vi "Autonomous Independent.vi"() -> ()   [LabVIEW 2014]
doc: "This VI is called when autonomous begins, and will automatically be terminated when autonomous ends. You can carry out timed or sensor driven robot movement independently without needing to return to the caller."
uses:
  Robot Global Data.vi
  <vilib>/Rock Robotics/WPI/Solenoid/Deprecated/WPI_SolenoidSetBool.vi
  <vilib>/Rock Robotics/WPI/DriverStation/DriverStationLCD/WPI_DriverStationLCDLCDLine.ctl
  <vilib>/Rock Robotics/SystemInterfaces/Typedef/FPGA_TypedefAnalogModule.ctl
  <vilib>/Rock Robotics/SystemInterfaces/AI/FPGA_AIChannel.ctl
  <vilib>/Rock Robotics/WPI/Gyro/WPI_GyroDevRef.ctl
panel:
  out "Boolean":bool
  in  "error in (no error)":errorcluster
  in  "GyroDevRef":T1={"DevStatus"={"status"=FALSE, "code"=0, "source"=""}, "Analog Module"=enum."Controller 1", "Analog Channel"=enum."AI 1", "Offset"=0.0, "Gain (VoltsPerDegree/Second)"=0.0}
  out "Gyro":dbl=111.9833474371419
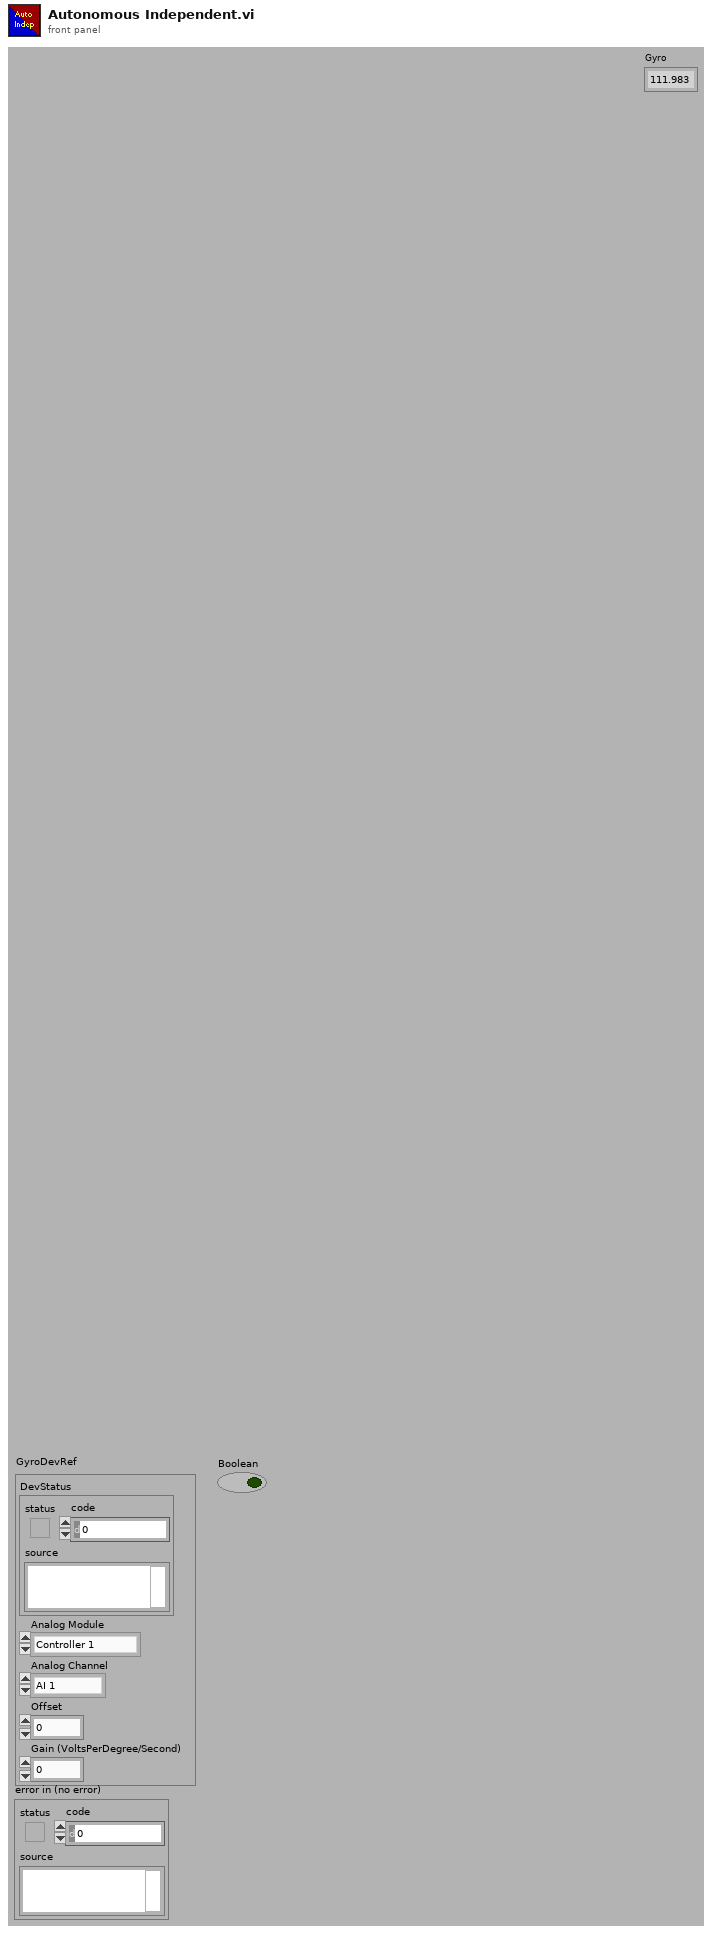
[diagram p1: front panel]
types:
  T1 = typedef "WPI_GyroDevRef.ctl" = cluster{"DevStatus":errorcluster, "Analog Module":T2, "Analog Channel":T3, "Offset":dbl, "Gain (VoltsPerDegree/Second)":dbl}
  T2 = typedef "FPGA_TypedefAnalogModule.ctl" = enum16{"Controller 1"}
  T3 = typedef "FPGA_AIChannel.ctl" = enum8{"AI 0", "AI 1", "AI 2", "AI 3", "AI MXP 0", "AI MXP 1", "AI MXP 2", "AI MXP 3", "Invalid"}
  T4 = typedef "WPI_DriverStationLCDLCDLine.ctl" = enum16{"Main - Line 1", "User - Line 2", "User - Line 3", "User - Line 4", "User - Line 5", "User - Line 6"}
  T5 = cluster{"Digital Input [1-16][0]":bool, "Digital Input [1-16][1]":bool, "Digital Input [1-16][2]":bool, "Digital Input [1-16][3]":bool, "Digital Input [1-16][4]":bool, "Digital Input [1-16][5]":bool, "Digital Input [1-16][6]":bool, "Digital Input [1-16][7]":bool, "Digital Input [1-16][8]":bool, "Digital Input [1-16][9]":bool, "Digital Input [1-16][10]":bool, "Digital Input [1-16][11]":bool, "Digital Input [1-16][12]":bool, "Digital Input [1-16][13]":bool, "Digital Input [1-16][14]":bool, "Digital Input [1-16][15]":bool}
  T6 = typedef "WPI_GyroDevRef.ctl" = cluster{"DevStatus":errorcluster, "Analog Module":T7, "Analog Channel":T8, "Offset":dbl, "Gain (VoltsPerDegree/Second)":dbl}
  T7 = typedef "FPGA_TypedefAnalogModule.ctl" = enum16{"Analog Module 1", "Analog Module 2"}
  T8 = typedef "FPGA_AIChannel.ctl" = enum8{"AI 1", "AI 2", "AI 3", "AI 4", "AI 5", "AI 6", "AI 7", "AI 8", "Invalid"}
  T9 = typedef "WPI_SolenoidDevRef.ctl" = cluster{"DevStatus":errorcluster, "Solenoid Module":T10, "Forward Solenoid Channel":T11, "Reverse Solenoid Channel":T11}
  T10 = typedef "FPGA_TypedefSolenoidModule.ctl" = enum16{"Solenoid Module 1", "Solenoid Module 2"}
  T11 = typedef "WPI_SolenoidChannel.ctl" = enum8{"Solenoid 1", "Solenoid 2", "Solenoid 3", "Solenoid 4", "Solenoid 5", "Solenoid 6", "Solenoid 7", "Solenoid 8", "Invalid"}
  T12 = typedef "WPI_EncoderDevRef.ctl" = cluster{"DevStatus":errorcluster, "EncoderIndex":T13, "CounterIndex":T14, "DistancePerCount":dbl, "Decoding Type":T15}
  T13 = typedef "FPGA_EncoderIdx.ctl" = enum8{"Enc 0", "Enc 1", "Enc 2", "Enc 3", "Invalid"}
  T14 = typedef "FPGA_CounterCtrSystemIndex.ctl" = enum8{"Ctr 0", "Ctr 1", "Ctr 2", "Ctr 3", "Ctr 4", "Ctr 5", "Ctr 6", "Ctr 7", "Invalid"}
  T15 = typedef "WPI_EncoderType.ctl" = enum16{"1x", "2x", "4x"}
  T16 = typedef "WPI_JoystickDevRef.ctl" = cluster{"Device":T17}
  T17 = typedef "WPI_JoystickDeviceEnum.ctl" = enum16{"USB 1", "USB 2", "USB 3", "USB 4", "Kinect 1", "Kinect 2"}
  T18 = typedef "WPI_JoystickButtonState.ctl" = cluster{"Button 1":bool, "Button 2":bool, "Button 3":bool, "Button 4":bool, "Button 5":bool, "Button 6":bool, "Button 7":bool, "Button 8":bool, "Button 9":bool, "Button 10":bool, "Button 11":bool, "Button 12":bool}
  T19 = typedef "WPI_DigitalInputDevRef.ctl" = cluster{"DevStatus":errorcluster, "DIO Channel":T20, "Digital Module":T21}
  T20 = typedef "FPGA_DIOChannel.ctl" = enum8{"DIO 1", "DIO 2", "DIO 3", "DIO 4", "DIO 5", "DIO 6", "DIO 7", "DIO 8", "DIO 9", "DIO 10", "DIO 11", "DIO 12", "DIO 13", "DIO 14", "Invalid"}
  T21 = typedef "FPGA_TypedefDigitalModule.ctl" = enum16{"Digital Module 1", "Digital Module 2"}
  T22 = typedef "WPI_RobotDriveDevRef.ctl" = cluster{"DevStatus":errorcluster, "Motors[]":T23[], "Square Inputs":bool, "Max Output":dbl, "Isochronous":bool}
  T23 = typedef "WPI_MotorControlDeviceRef.ctl" = cluster{"DeviceStatus":errorcluster, "Type":enum16{"PWM", "CAN"}, "PWM":cluster{"Digital Module":T21, "PWM Channel":T24, "DeadBand":T25}, "CAN":cluster{"Device Number":u8, "Control Mode":T26, "Semaphore":T27, "Max Vout":dbl}, "Invert":bool, "TransformRef":T28, "InvTransformRef":T28}
  T24 = typedef "FPGA_DIOPWMChannel.ctl" = enum8{"PWM 1", "PWM 2", "PWM 3", "PWM 4", "PWM 5", "PWM 6", "PWM 7", "PWM 8", "PWM 9", "PWM 10", "Invalid"}
  T25 = typedef "WPI_PWMDeadband.ctl" = cluster{"Name":string, "maxPositivePwm":i32, "minPositivePwm":i32, "centerPwm":i32, "maxNegativePwm":i32, "minNegativePwm":i32, "angularRange":u16}
  T26 = typedef "WPI_CANJaguar_ControlMode.ctl" = enum8{"Percent VBus", "Current", "Speed", "Position", "Voltage"}
  T27 = typedef "Semaphore RefNum" = refnum<k1>
  T28 = typedef "WPI_PWMTransform_ConPane.ctl" = refnum<vi>
  T29 = cluster{"axis 1 (x)":dbl, "axis 2 (y)":dbl, "axis 3 (throttle)":dbl, "axis 4":dbl, "axis 5":dbl, "axis 6":dbl}
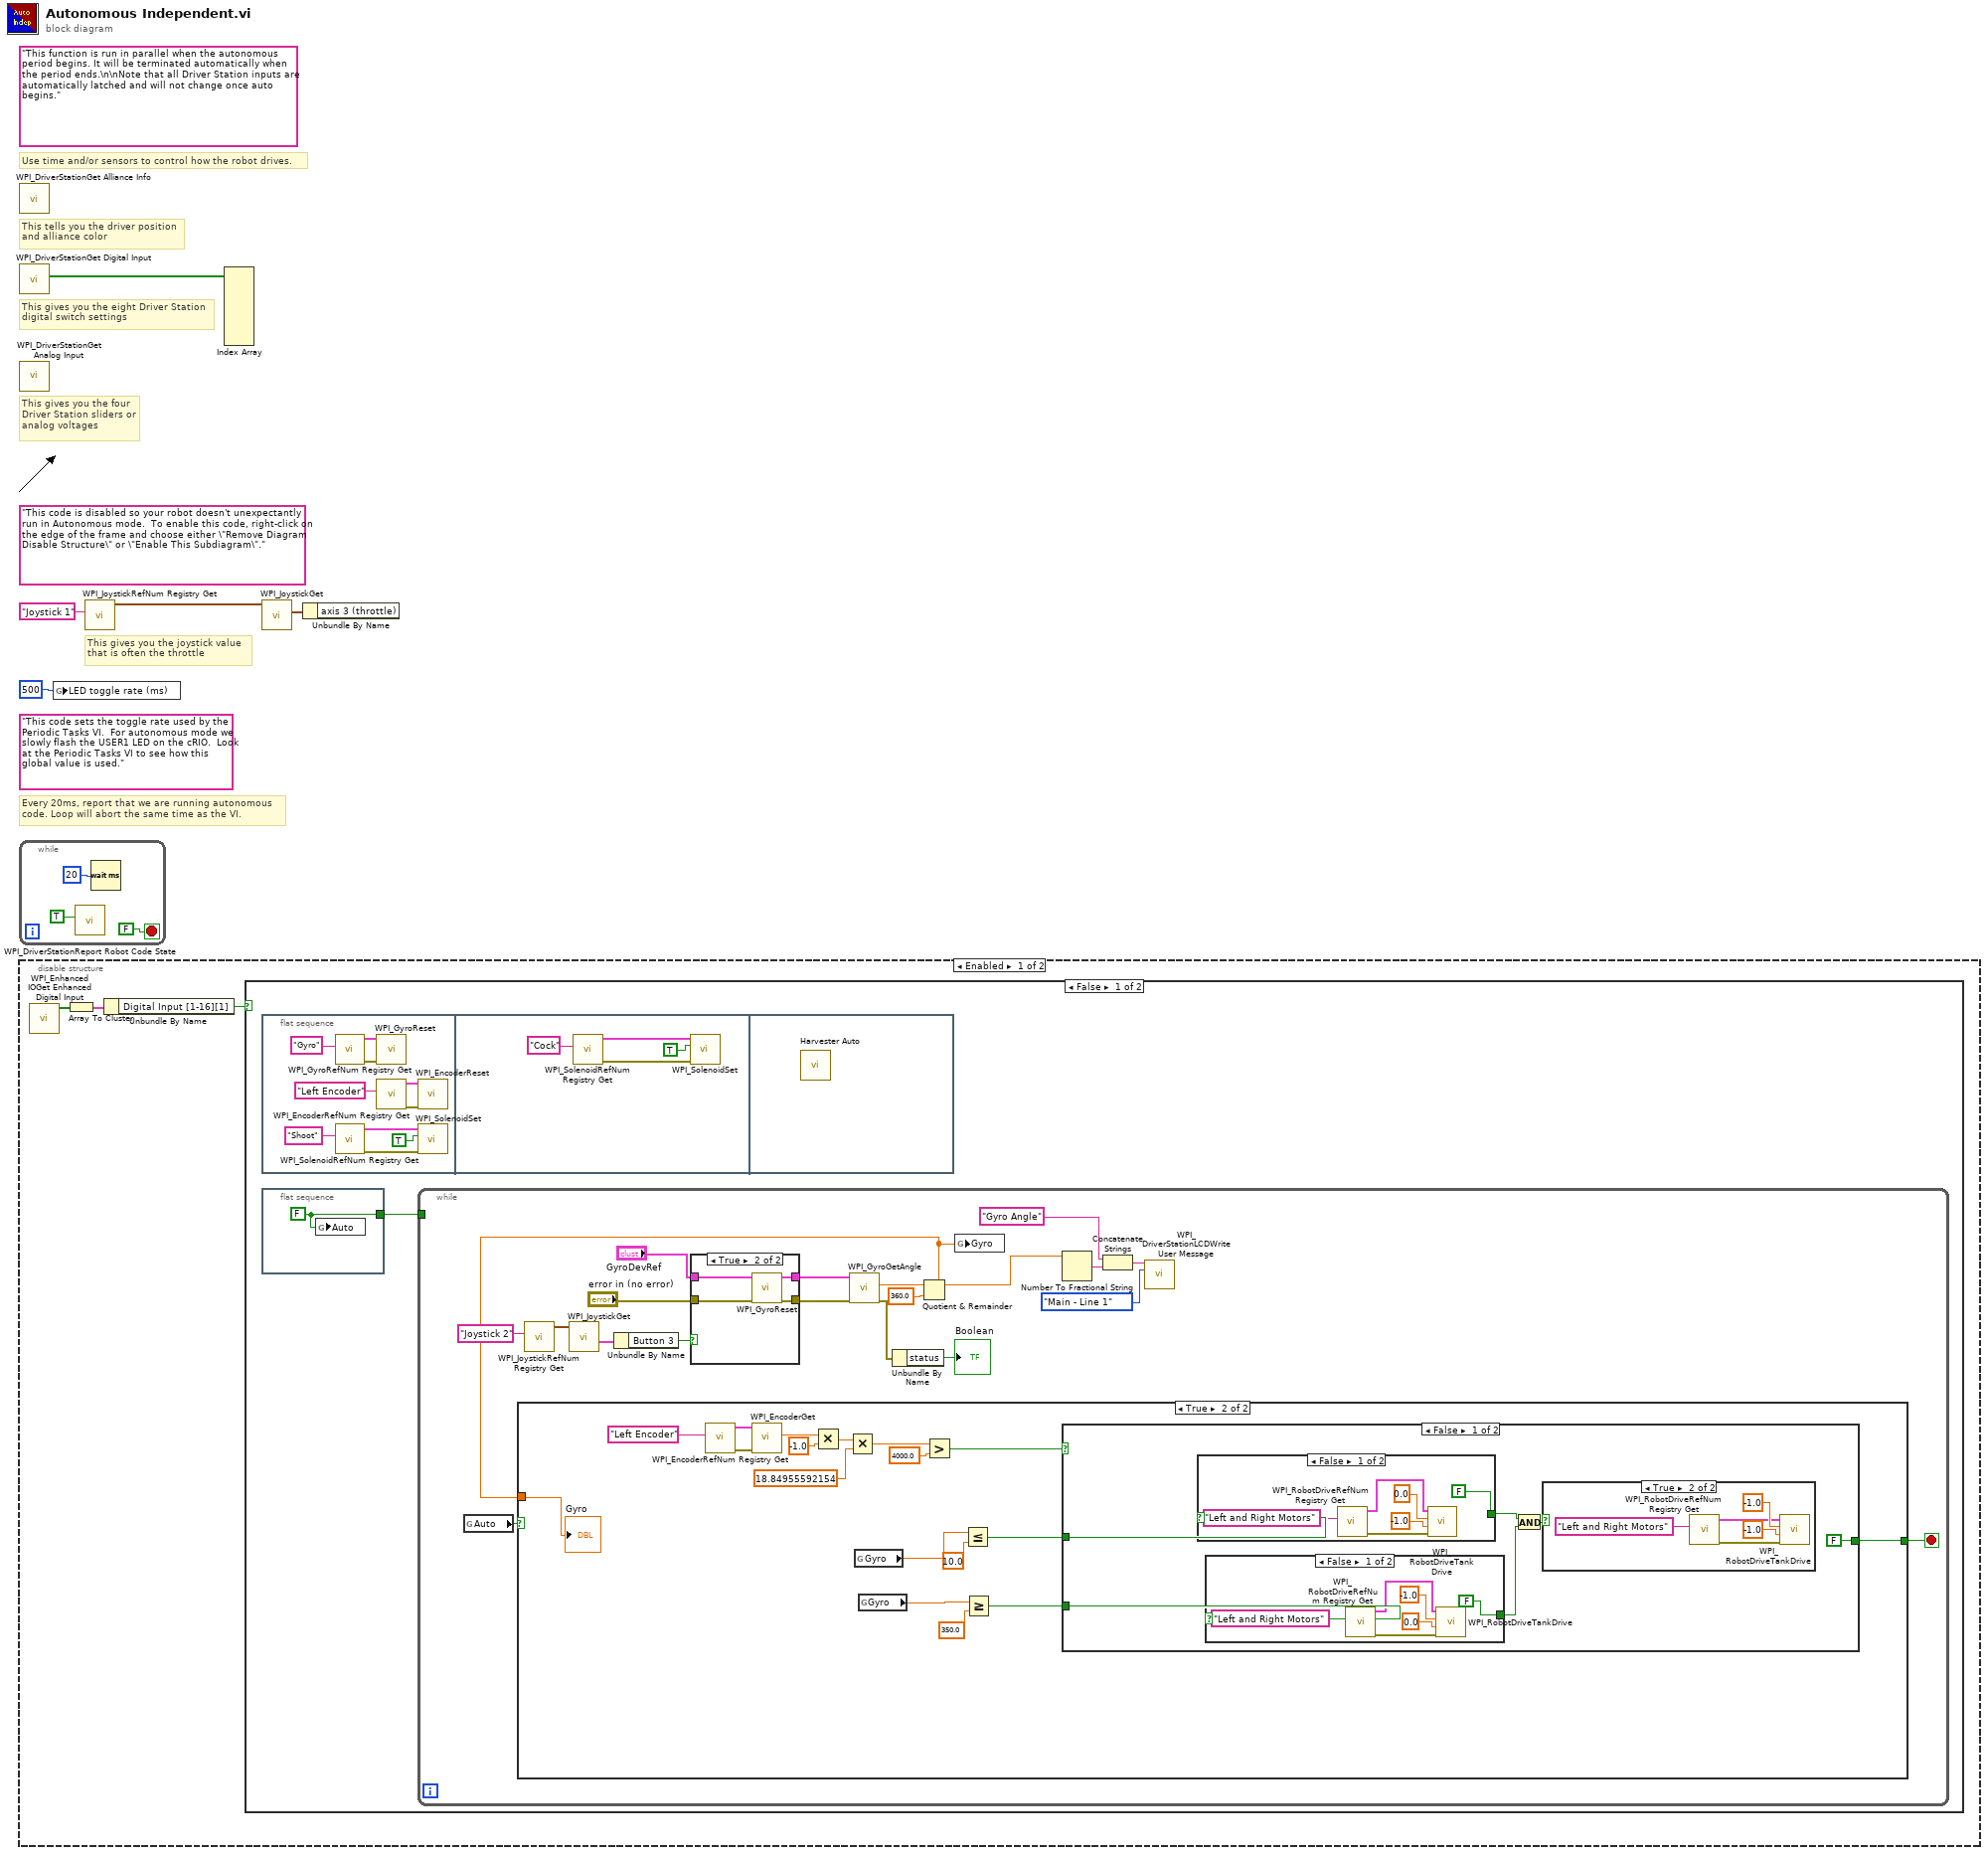
[diagram p0: block diagram]
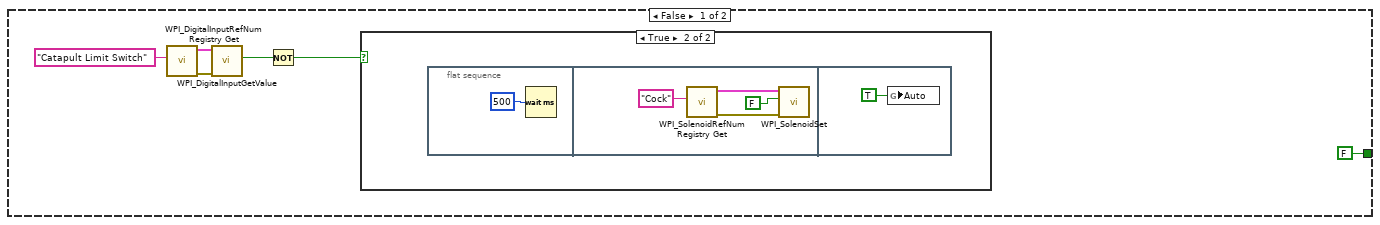
[diagram p3: hidden frame]
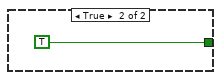
[diagram p6: hidden frame]
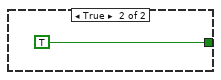
[diagram p7: hidden frame]
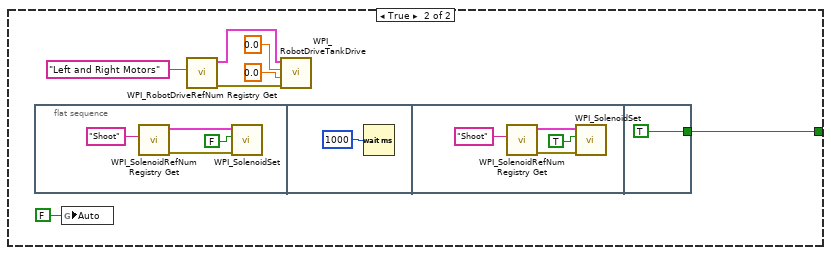
[diagram p8: hidden frame]
diagram:
  (unwired) "This code sets the toggle rate used by the Periodic Tasks VI.  For autonomous mode we slowly flash the USER1 LED on the cRIO.  Look at the Periodic Tasks VI to see how this global value is used."
  (unwired) "This code is disabled so your robot doesn't unexpectantly run in Autonomous mode.  To enable this code, right-click on the edge of the frame and choose either \"Remove Diagram Disable Structure\" or \"Enable This Subdiagram\"."
  (unwired) "This function is run in parallel when the autonomous period begins. It will be terminated automatically when the period ends.\n\nNote that all Driver Station inputs are automatically latched and will not change once auto begins."
  # "Every 20ms, report that we are running autonomous\ncode. Loop will abort the same time as the VI."
  # "This gives you the joystick value\nthat is often the throttle"
  # "Use time and/or sensors to control how the robot drives."
  # "This tells you the driver position\nand alliance color"
  # "This gives you the eight Driver Station\ndigital switch settings"
  # "This gives you the four\nDriver Station sliders or\nanalog voltages"
  n1 = call <vilib>:"WPI_DriverStationGet Alliance Info.vi"() -> ()  [unwired: 12 out]
  n2 = call <vilib>:"WPI_DriverStationGet Digital Input.vi"() -> ("Driver Station Digital Input (1-8)"=w5:bool[])  [unwired: 11 out]
  n3 = call <vilib>:"WPI_DriverStationGet Analog Input.vi"() -> ()  [unwired: 12 out]
  n4 = while {
    stop <- FALSE stop-if-true
    n5 = call <vilib>:"WPI_DriverStationReport Robot Code State.vi"("Autonomous"=TRUE) -> ()  [unwired: 10 in, 1 out]
    n6 = Wait (ms)(milliseconds to wait=u32 20) -> ()  [unwired: 1 out]
  }
  n7 = disable-structure shown="Enabled" {
    frame Enabled {
      n8 = call <vilib>:"WPI_Enhanced IOGet Enhanced Digital Input.vi"() -> ("Digital Input [1-16]"=w11:bool[])  [unwired: 10 in, 1 out]
      n9 = Array To Cluster(array=w11) -> (cluster=w10:T5)
      n10 = Unbundle By Name(w10) -> ("Digital Input [1-16][1]"=w9:bool)
      n11 = case shown="False" w9 {
        frame False {
          n12 = flat-sequence {
            frame #0 {
              n13 = call <vilib>:"WPI_GyroRefNum Registry Get.vi"("refnum name"="Gyro") -> ("error out"=w112:errorcluster, "GyroDevRef"=w113:T6)  [unwired: 9 in]
              n14 = call <vilib>:"WPI_SolenoidRefNum Registry Get.vi"("refnum name"="Shoot") -> ("error out"=w114:errorcluster, "SolenoidDevRef"=w115:T9)  [unwired: 9 in]
              n15 = call <vilib>:"WPI_GyroReset.vi"("error in (no error)"=w112, "GyroDevRef"=w113) -> ()  [unwired: 10 out]
              n16 = call <vilib>:"WPI_EncoderRefNum Registry Get.vi"("refnum name"="Left Encoder") -> ("error out"=w120:errorcluster, "EncoderDevRef"=w119:T12)  [unwired: 9 in]
              n17 = call <vilib>:"WPI_EncoderReset.vi"("error in (no error)"=w120, "EncoderDevRef"=w119) -> ()  [unwired: 8 in, 2 out]
              n18 = call-poly <vilib>:"WPI_SolenoidSet.vi"("error in (no error)"=w114, "Value"=TRUE, "SolenoidDevRef"=w115) -> ()  [unwired: 7 in, 2 out]
            }
            frame #1 {
              n19 = call <vilib>:"WPI_SolenoidRefNum Registry Get.vi"("refnum name"="Cock") -> ("error out"=w124:errorcluster, "SolenoidDevRef"=w122:T9)  [unwired: 9 in]
              n20 = call-poly <vilib>:"WPI_SolenoidSet.vi"("error in (no error)"=w124, "Value"=TRUE, "SolenoidDevRef"=w122) -> ()  [unwired: 7 in, 2 out]
            }
            frame #2 {
              n21 = call "Harvester Auto.vi"() -> ()  [unwired: 12 in]
            }
          }
          n22 = flat-sequence {
            tunnel: [w13] -> w12
            frame #0 {
              w13 = FALSE
              n23 = global write "Robot Global Data.vi" "Auto"(w13) -> ()
            }
          }
          n24 = while {
            tunnel: w12 -> [_]
            stop <- w31 stop-if-true
            n25 = global read "Robot Global Data.vi" "Auto"() -> (w32:bool)
            n26 = call <vilib>:"WPI_JoystickRefNum Registry Get.vi"("refnum name"="Joystick 2") -> ("JoystickDevRef"=w28:T16)  [unwired: 1 in, 9 out]
            n27 = call <vilib>:"WPI_JoystickGet.vi"("JoystickDevRef"=w28) -> ("Buttons"=w29:T18)  [unwired: 1 in, 5 out]
            n28 = Unbundle By Name(w29) -> ("Button 3"=w30:bool)
            n29 = case shown="True" w30 {
              tunnel: [w34 w38] -> w20
              tunnel: [w33 w37] -> w23
              tunnel: "GyroDevRef" -> [w34 w36]
              tunnel: "error in (no error)" -> [w33 w35]
              frame False {
              }
              frame True {
                n30 = call <vilib>:"WPI_GyroReset.vi"("error in (no error)"=w35, "GyroDevRef"=w36) -> ("error out"=w37:errorcluster, "GyroDevRef"=w38:T6)  [unwired: 8 out]
              }
            }
            n31 = call <vilib>:"WPI_GyroGetAngle.vi"("error in (no error)"=w23, "GyroDevRef"=w20) -> ("error out"=w21:errorcluster, "Angle"=w16:dbl)  [unwired: 8 out]
            n32 = Unbundle By Name(w21) -> ("status"=→"Boolean":bool)
            n33 = Quotient & Remainder(x=w16, y=360.0) -> (x-y*floor(x/y)=w14:dbl)  [unwired: 1 out]
            n34 = case shown="True" w32 {
              tunnel: [FALSE w59] -> w31
              tunnel: w14 -> [_ w57]
              frame False {
                n35 = call <vilib>:"WPI_DigitalInputRefNum Registry Get.vi"("refnum name"="Catapult Limit Switch") -> ("error out"=w40:errorcluster, "DigitalInputDevRef"=w41:T19)  [unwired: 9 in]
                n36 = call <vilib>:"WPI_DigitalInputGetValue.vi"("error in (no error)"=w40, "DigitalInputDevRef"=w41) -> ("Value"=w43:bool)  [unwired: 7 in, 2 out]
                n37 = Not(x=w43) -> (.not. x?=w42:bool)
                n38 = case shown="True" w42 {
                  frame False {
                  }
                  frame True {
                    n39 = flat-sequence {
                      frame #0 {
                        n40 = Wait (ms)(milliseconds to wait=u32 500) -> ()  [unwired: 1 out]
                      }
                      frame #1 {
                        n41 = call <vilib>:"WPI_SolenoidRefNum Registry Get.vi"("refnum name"="Cock") -> ("error out"=w46:errorcluster, "SolenoidDevRef"=w47:T9)  [unwired: 9 in]
                        n42 = call-poly <vilib>:"WPI_SolenoidSet.vi"("error in (no error)"=w46, "Value"=FALSE, "SolenoidDevRef"=w47) -> ()  [unwired: 7 in, 2 out]
                      }
                      frame #2 {
                        n43 = global write "Robot Global Data.vi" "Auto"(TRUE) -> ()
                      }
                    }
                  }
                }
              }
              frame True {
                n44 = call <vilib>:"WPI_EncoderRefNum Registry Get.vi"("refnum name"="Left Encoder") -> ("error out"=w62:errorcluster, "EncoderDevRef"=w61:T12)  [unwired: 9 in]
                n45 = call <vilib>:"WPI_EncoderGet.vi"("error in (no error)"=w62, "EncoderDevRef"=w61) -> ("Distance"=w64:dbl)  [unwired: 4 in, 5 out]
                n46 = Multiply(x=w64, y=-1.0) -> (x*y=w63:dbl)
                n47 = Multiply(x=w63, y=18.84955592154) -> (x*y=w60:dbl)
                n48 = global read "Robot Global Data.vi" "Gyro"() -> (w55:dbl)
                n49 = global read "Robot Global Data.vi" "Gyro"() -> (w53:dbl)
                n50 = Greater?(x=w60, y=4000.0) -> (0:w58:bool)
                n51 = Less Or Equal?(x=w55, y=10.0) -> (x <= y?=w52:bool)
                n52 = Greater Or Equal?(x=w53, y=350.0) -> (x >= y?=w51:bool)
                n53 = case shown="False" w58 {
                  tunnel: [FALSE w94] -> w59
                  tunnel: w52 -> [w73 _]
                  tunnel: w51 -> [w72 _]
                  frame False {
                    n54 = case shown="False" w73 {
                      tunnel: [FALSE TRUE] -> w70
                      frame False {
                        n55 = call <vilib>:"WPI_RobotDriveRefNum Registry Get.vi"("refnum name"="Left and Right Motors") -> ("error out"=w88:errorcluster, "RobotDriveDevRef"=w89:T22)  [unwired: 9 in]
                        n56 = call <vilib>:"WPI_RobotDriveTankDrive.vi"("error in (no error)"=w88, "Right axis value"=-1.0 ("RightSpeed"), "Left axis value"=0.0 ("LeftSpeed"), "RobotDriveDevRef"=w89) -> ()  [unwired: 5 in, 3 out]
                      }
                      frame True {
                      }
                    }
                    n57 = case shown="False" w72 {
                      tunnel: [FALSE TRUE] -> w69
                      frame False {
                        n58 = call <vilib>:"WPI_RobotDriveRefNum Registry Get.vi"("refnum name"="Left and Right Motors") -> ("error out"=w81:errorcluster, "RobotDriveDevRef"=w82:T22)  [unwired: 9 in]
                        n59 = call <vilib>:"WPI_RobotDriveTankDrive.vi"("error in (no error)"=w81, "Right axis value"=0.0 ("RightSpeed"), "Left axis value"=-1.0 ("LeftSpeed"), "RobotDriveDevRef"=w82) -> ()  [unwired: 5 in, 3 out]
                      }
                      frame True {
                      }
                    }
                    n60 = And(x=w70, y=w69) -> (x .and. y?=w71:bool)
                    n61 = case shown="True" w71 {
                      frame False {
                      }
                      frame True {
                        n62 = call <vilib>:"WPI_RobotDriveRefNum Registry Get.vi"("refnum name"="Left and Right Motors") -> ("error out"=w75:errorcluster, "RobotDriveDevRef"=w76:T22)  [unwired: 9 in]
                        n63 = call <vilib>:"WPI_RobotDriveTankDrive.vi"("error in (no error)"=w75, "Right axis value"=-1.0 ("RightSpeed"), "Left axis value"=-1.0 ("LeftSpeed"), "RobotDriveDevRef"=w76) -> ()  [unwired: 5 in, 3 out]
                      }
                    }
                  }
                  frame True {
                    n64 = flat-sequence {
                      tunnel: [TRUE] -> w94
                      frame #0 {
                        n65 = call <vilib>:"WPI_SolenoidRefNum Registry Get.vi"("refnum name"="Shoot") -> ("error out"=w104:errorcluster, "SolenoidDevRef"=w101:T9)  [unwired: 9 in]
                        n66 = call-poly <vilib>:"WPI_SolenoidSet.vi"("error in (no error)"=w104, "Value"=FALSE, "SolenoidDevRef"=w101) -> ()  [unwired: 7 in, 2 out]
                      }
                      frame #1 {
                        n67 = Wait (ms)(milliseconds to wait=u32 1000) -> ()  [unwired: 1 out]
                      }
                      frame #2 {
                        n68 = call <vilib>:"WPI_SolenoidRefNum Registry Get.vi"("refnum name"="Shoot") -> ("error out"=w109:errorcluster, "SolenoidDevRef"=w108:T9)  [unwired: 9 in]
                        n69 = call-poly <vilib>:"WPI_SolenoidSet.vi"("error in (no error)"=w109, "Value"=TRUE, "SolenoidDevRef"=w108) -> ()  [unwired: 7 in, 2 out]
                      }
                      frame #3 {
                      }
                    }
                    n70 = global write "Robot Global Data.vi" "Auto"(FALSE) -> ()
                    n71 = call <vilib>:"WPI_RobotDriveRefNum Registry Get.vi"("refnum name"="Left and Right Motors") -> ("error out"=w96:errorcluster, "RobotDriveDevRef"=w97:T22)  [unwired: 9 in]
                    n72 = call <vilib>:"WPI_RobotDriveTankDrive.vi"("error in (no error)"=w96, "Right axis value"=0.0 ("RightSpeed"), "Left axis value"=0.0 ("LeftSpeed"), "RobotDriveDevRef"=w97) -> ()  [unwired: 5 in, 3 out]
                  }
                }
                "Gyro" <- w57
              }
            }
            n73 = global write "Robot Global Data.vi" "Gyro"(w14) -> ()
            n74 = Number To Fractional String(number=w14) -> (F-format string=w18:string)  [unwired: 3 out]
            n75 = Concatenate Strings("Gyro Angle" ("string"), w18) -> (w22:string)
            n76 = call <vilib>:"WPI_DriverStationLCDWrite User Message.vi"("line text"=w22, "line"=WPI_DriverStationLCDLCDLine."Main - Line 1") -> ()  [unwired: 3 in, 11 out]
          }
        }
        frame True {
        }
      }
    }
    frame Disabled {
    }
  }
  n77 = global write "Robot Global Data.vi" "LED toggle rate (ms)"(u32 500 ("LED ms toggle rate")) -> ()
  n78 = call <vilib>:"WPI_JoystickRefNum Registry Get.vi"("refnum name"="Joystick 1") -> ("JoystickDevRef"=w2:T16)  [unwired: 1 in, 9 out]
  n79 = Index Array(array=w5) -> ()  [unwired: 8 in, 8 out]
  n80 = call <vilib>:"WPI_JoystickGet.vi"("JoystickDevRef"=w2) -> ("Axes"=w3:T29)  [unwired: 1 in, 5 out]
  n81 = Unbundle By Name(w3) -> ()  [unwired: 1 out]
